vi "Poll All Sensors.vi"(8 "error in":errorcluster, 11 "UART port in":T9) -> (0 "error out":errorcluster, 1 "Timed Out?":bool, 2 "iRobot Sensors":T1={"Bumps + Wheel Drops"={"Wheeldrop Caster"=FALSE, "Wheeldrop Left"=FALSE, "Wheeldrop Right"=FALSE, "Bump Left"=FALSE, "Bump Right"=FALSE}, "Wall"=FALSE, "Cliff Left"=FALSE, "Cliff Front Left"=FALSE, "Cliff Front Right"=FALSE, "Cliff Right"=FALSE, "Virtual Wall"=FALSE, "Low-Side Driver + Wheel Overcurrent"={"Low-Side Driver 0"=FALSE, "Low-Side Driver 1"=FALSE, "Low-Side Driver 2"=FALSE, "Left Wheel"=FALSE, "Right Wheel"=FALSE}, "Infrared"=255, "Buttons"={"Advance"=FALSE, "Play"=FALSE}, "Distance (mm)"=0, "Angle (deg)"=0, "Charging State"=enum."Not Charging", "Voltage (mV)"=0, "Current (mA)"=0, "Battery Temperature (deg C)"=0, "Battery Charge (mAh)"=0, "Battery Capacity (mAh)"=0, "Wall Signal (0-4095)"=0, "Cliff Left Signal (0-4095)"=0, "Cliff Front Left Signal (0-4095)"=0, "Cliff Front Right Signal (0-4095)"=0, "Cliff Right Signal (0-4095)"=0, "Cargo Bay Digital Inputs"={"Digital Input 0"=FALSE, "Digital Input 1"=FALSE, "Digital Input 2"=FALSE, "Digital Input 3"=FALSE, "Device Detect"=FALSE}, "Cargo Bay Analog Signal (0-1023)"=0, "Charging Sources Available"={"Internal Charger"=FALSE, "Home Base"=FALSE}, "OI Mode"=enum."Off", "Song Number"=0, "Song Playing"=FALSE, "Number of Stream Packets"=0, "Requested Velocity (mm/s)"=0, "Requested Radius (mm)"=0, "Requested Right Wheel Velocity (mm/s)"=0, "Requested Left Wheel Velocity (mm/s)"=0} {"Infrared" format="%02x"}, 3 "UART port out":T9)   [LabVIEW 2015]
doc: "Polls the iRobot Create for Sensor Group 6 (all sensors).\n\nDo not call this VI if a sensor stream has been configured; instead, use streaming VIs.\n\nThis VI both writes to AND reads from the serial port\n<b>NOTE</b>: This should not be used in a loop if other serial reading or writing VIs are called in parallel loops."
uses:
  Advanced/UART/iRobot UART Port Type.ctl
  Sensor Group 6.ctl
  Bumps + Wheel Drops.ctl
  Low-Side Driver + Wheel Overcurrent.ctl
  Buttons.ctl
  Charging State.ctl
  Cargo Bay Digital Inputs.ctl
  Charging Sources Available.ctl
  OI Mode.ctl
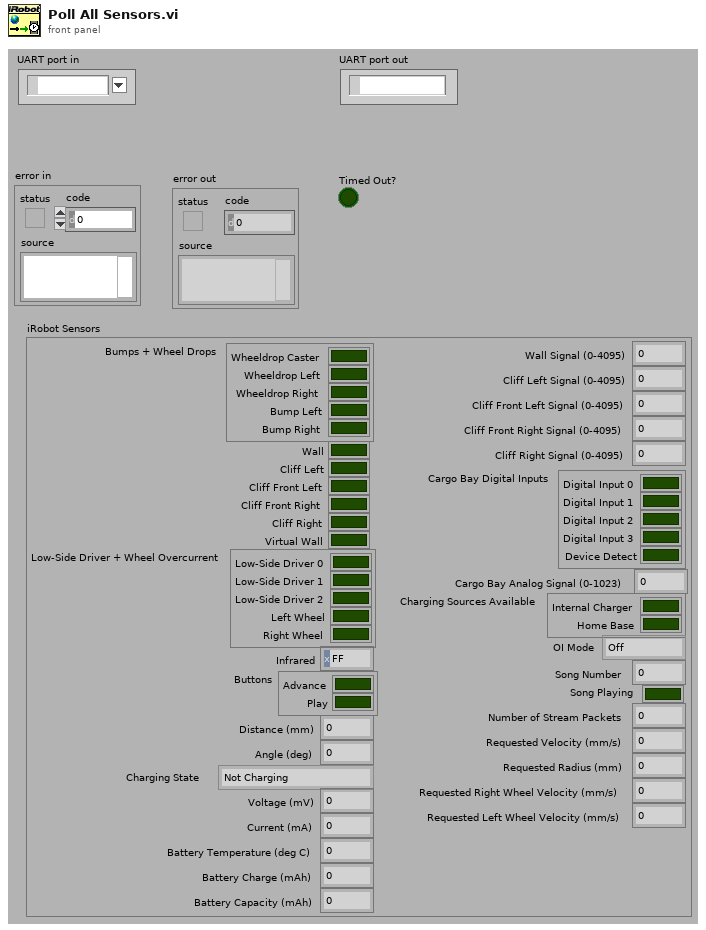
[diagram p1: front panel]
types:
  T1 = typedef "Sensor Group 6.ctl" = cluster{"Bumps + Wheel Drops":T2, "Wall":bool, "Cliff Left":bool, "Cliff Front Left":bool, "Cliff Front Right":bool, "Cliff Right":bool, "Virtual Wall":bool, "Low-Side Driver + Wheel Overcurrent":T3, "Infrared":u8, "Buttons":T4, "Distance (mm)":i32, "Angle (deg)":i32, "Charging State":T5, "Voltage (mV)":u16, "Current (mA)":i16, "Battery Temperature (deg C)":i8, "Battery Charge (mAh)":u16, "Battery Capacity (mAh)":u16, "Wall Signal (0-4095)":u16, "Cliff Left Signal (0-4095)":u16, "Cliff Front Left Signal (0-4095)":u16, "Cliff Front Right Signal (0-4095)":u16, "Cliff Right Signal (0-4095)":u16, "Cargo Bay Digital Inputs":T6, "Cargo Bay Analog Signal (0-1023)":u16, "Charging Sources Available":T7, "OI Mode":T8, "Song Number":u8, "Song Playing":bool, "Number of Stream Packets":u8, "Requested Velocity (mm/s)":i16, "Requested Radius (mm)":i16, "Requested Right Wheel Velocity (mm/s)":i16, "Requested Left Wheel Velocity (mm/s)":i16}
  T2 = typedef "Bumps + Wheel Drops.ctl" = cluster{"Wheeldrop Caster":bool, "Wheeldrop Left":bool, "Wheeldrop Right":bool, "Bump Left":bool, "Bump Right":bool}
  T3 = typedef "Low-Side Driver + Wheel Overcurrent.ctl" = cluster{"Low-Side Driver 0":bool, "Low-Side Driver 1":bool, "Low-Side Driver 2":bool, "Left Wheel":bool, "Right Wheel":bool}
  T4 = typedef "Buttons.ctl" = cluster{"Advance":bool, "Play":bool}
  T5 = typedef "Charging State.ctl" = enum16{"Not Charging", "Reconditioning Charging", "Full Charging", "Trickle Charging", "Waiting", "Charging Fault Condition"}
  T6 = typedef "Cargo Bay Digital Inputs.ctl" = cluster{"Digital Input 0":bool, "Digital Input 1":bool, "Digital Input 2":bool, "Digital Input 3":bool, "Device Detect":bool}
  T7 = typedef "Charging Sources Available.ctl" = cluster{"Internal Charger":bool, "Home Base":bool}
  T8 = typedef "OI Mode.ctl" = enum16{"Off", "Passive", "Safe", "Full"}
  T9 = typedef "iRobot UART Port Type.ctl" = refnum<visa-resource-name>
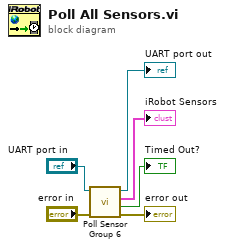
[diagram p0: block diagram]
diagram:
  n1 = call "Poll Sensor Group 6.vi"("error in"="error in", "UART port in"="UART port in") -> ("error out"=→"error out":errorcluster, "Timed Out?"=→"Timed Out?":bool, "iRobot Sensor Group 6"=→"iRobot Sensors":T1, "UART port out"=→"UART port out":T9)  [unwired: 6 in]
